vi "GetParam.vi"(8 "error in (no error)":errorcluster caption="entrée d'erreur (pas d'erreur)", 11 "StandardScaler.lvclass":refnum<class "StandardScaler.lvclass">) -> (0 "error out":errorcluster caption="sortie d'erreur", 2 "StandardScaler":T1={"copy"=TRUE, "with_mean"=TRUE, "with_std"=TRUE}, 3 "StandardScaler.lvclass":refnum<class "StandardScaler.lvclass">)   [LabVIEW 2020, in "StandardScaler.lvclass"]
doc: "Get Parameters"
uses:
  StandardScaler.lvclass
  StandardScaler.lvclass/StandardScaler.ctl
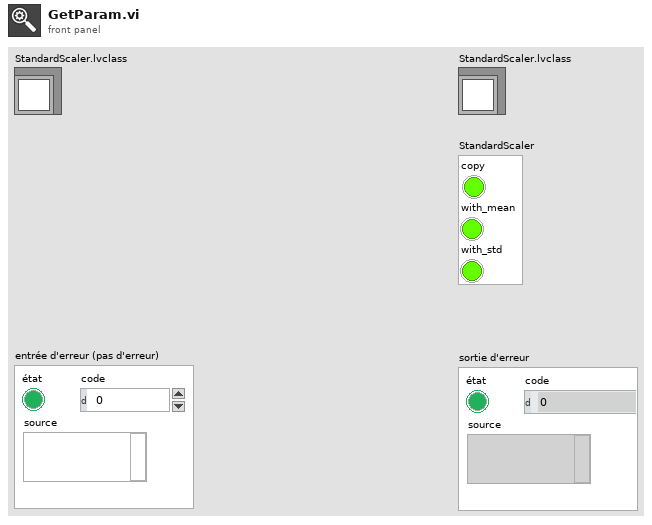
[diagram p1: front panel]
types:
  T1 = cluster{"copy":bool, "with_mean":bool, "with_std":bool}
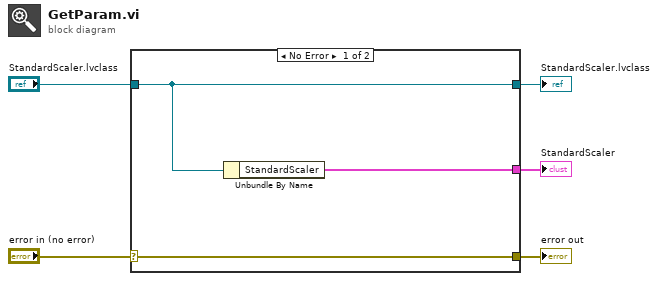
[diagram p0: block diagram]
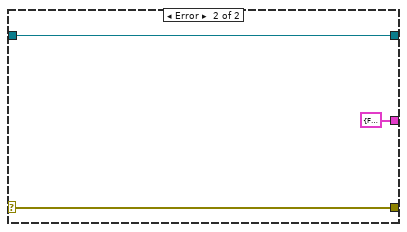
[diagram p2: hidden frame]
diagram:
  n1 = case shown="No Error" "error in (no error)" {
    selector: "error in (no error)" -> [w8 w10]
    tunnel: [w8 w10] -> w4
    tunnel: [w7 w11] -> w2
    tunnel: "StandardScaler.lvclass" -> [w7 w11]
    tunnel: [w6 T1 {"copy"=FALSE, "with_mean"=FALSE, "with_std"=FALSE} ("StandardScaler")] -> w1
    frame No Error {
      n2 = Unbundle By Name(w7) -> ("StandardScaler"=w6:T1)
    }
    frame Error {
    }
  }
  "error out" <- w4
  "StandardScaler.lvclass" <- w2
  "StandardScaler" <- w1
